vi "SetupCallBackEvents.vi"(8 "error in (no error)":errorcluster, 11 "DataGridView in":refnum<class "DataGridView.lvclass">) -> (0 "error out":errorcluster, 3 "DataGridView out":refnum<class "DataGridView.lvclass">)   [LabVIEW 2014, in "DataGridView.lvclass"]
uses:
  DataGridView.lvclass
  DataGridView.lvclass/DataGridView.ctl
  Read DataGridView.vi
  System.Windows.Forms
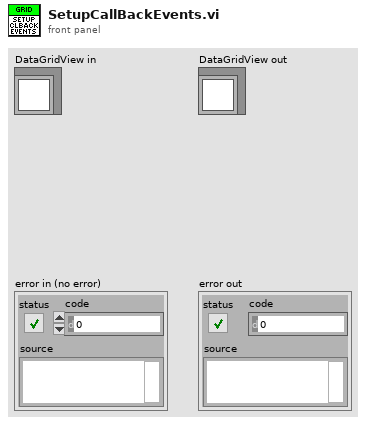
[diagram p1: front panel]
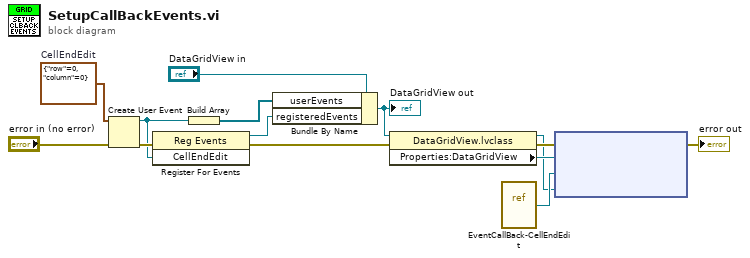
[diagram p0: block diagram]
diagram:
  w13 = cluster{"row":i32, "column":i32} {"row"=0, "column"=0}  # CellEndEdit
  n1 = Create User Event(user event datatype=w13, error in="error in (no error)") -> (user event=w12:refnum<user-event>, error out=w14:errorcluster)
  n2 = register-events(error in=w14, w12) -> (reference out=w4:refnum<event-registration>, error out=w3:errorcluster)  [unwired: 1 in]
  n3 = Build Array(w12) -> (w5:refnum<user-event>[])
  n4 = Bundle By Name(cluster="DataGridView in", "userEvents"=w5, "registeredEvents"=w4) -> (w1:refnum<class "DataGridView.lvclass">)
  "DataGridView out" <- w1
  n5 = property class="DataGridView.lvclass"(reference=w1, error in=w3) -> (reference out=w8:refnum<class "DataGridView.lvclass">, error out=w9:errorcluster, "Properties:DataGridView"=w10:refnum<k24>)
  n6 = vi-ref "EventCallBack-CellEndEdit.vi"() -> ("vi reference"=w11:refnum<vi>)
  n7 = node(w9, w10, w11, w8) -> (→"error out":errorcluster)  [unwired: 1 in, 1 out]
